vi "Get Route Distance.vi"(8 "Error In":errorcluster, 11 "ROute Index":i32) -> (0 "error out":errorcluster, 3 "Distance":dbl)   [LabVIEW 2014]
uses:
  C:/Robotic Systems/Products/AgFalcon/Software/Ground Station/Data/Mapping DLL/GMap.NET.WindowsForms.dll
  Data/Mapping DLL/GMap.NET.WindowsForms.dll
  Reference/SubVI/Main Map Control Refernce.vi
  Missions/FGVs/Current Mission Distance/Methods/Set Mission Distance.vi
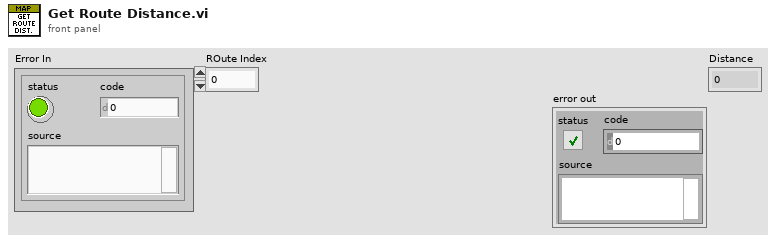
[diagram p1: front panel]
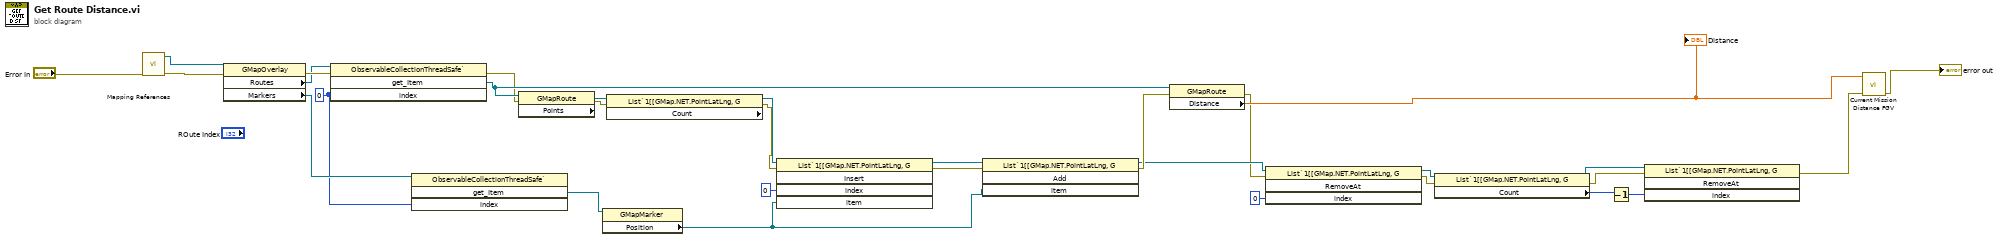
[diagram p0: block diagram]
diagram:
  w14 = 0 ("index")
  n1 = call-poly "Mapping References.vi"("Error In"="Error In") -> ("Error Out"=w30:errorcluster, "Main Map Reference"=w28:refnum<k24>)  [unwired: 9 in]
  n2 = property class="GMapOverlay"(reference=w28, error in=w30) -> (error out=w31:errorcluster, "Routes"=w29:refnum<k24>, "Markers"=w15:refnum<k24>)  [unwired: 1 out]
  n3 = invoke class="ObservableCollectionThreadSafe`" method="get_Item"(reference=w29, error in=w31, "index"=w14) -> (error out=w24:errorcluster, "get_Item"=w26:refnum<k24>)  [unwired: 1 in, 2 out]
  n4 = invoke class="ObservableCollectionThreadSafe`" method="get_Item"(reference=w15, "index"=w14) -> ("get_Item"=w13:refnum<k24>)  [unwired: 2 in, 3 out]
  n5 = property class="GMapRoute"(reference=w26, error in=w24) -> (error out=w23:errorcluster, "Points"=w25:refnum<k24>)  [unwired: 1 out]
  n6 = property class="GMapMarker"(reference=w13) -> ("Position"=w7:refnum<k24>)  [unwired: 1 in, 2 out]
  n7 = property class="List`1[[GMap.NET.PointLatLng, G" props=["Count"](reference=w25, error in=w23) -> (reference out=w20:refnum<k24>, error out=w16:errorcluster)  [unwired: 1 out]
  n8 = invoke class="List`1[[GMap.NET.PointLatLng, G" method="Insert"(reference=w20, error in=w16, "index"=0, "item"=w7) -> (reference out=w18:refnum<k24>, error out=w17:errorcluster)  [unwired: 1 in, 3 out]
  n9 = invoke class="List`1[[GMap.NET.PointLatLng, G" method="Add"(reference=w18, error in=w17, "item"=w7) -> (reference out=w11:refnum<k24>, error out=w12:errorcluster)  [unwired: 1 in, 2 out]
  n10 = property class="GMapRoute"(reference=w26, error in=w12) -> (error out=w10:errorcluster, "Distance"=w22:dbl)  [unwired: 1 out]
  "Distance" <- w22
  n11 = invoke class="List`1[[GMap.NET.PointLatLng, G" method="RemoveAt"(reference=w11, error in=w10, "index"=0) -> (reference out=w6:refnum<k24>, error out=w5:errorcluster)  [unwired: 1 in, 2 out]
  n12 = property class="List`1[[GMap.NET.PointLatLng, G"(reference=w6, error in=w5) -> (reference out=w1:refnum<k24>, error out=w2:errorcluster, "Count"=w4:i32)
  n13 = Decrement(x=w4) -> (x-1=w3:i32)
  n14 = invoke class="List`1[[GMap.NET.PointLatLng, G" method="RemoveAt"(reference=w1, error in=w2, "index"=w3) -> (error out=w9:errorcluster)  [unwired: 1 in, 3 out]
  n15 = call-poly "Current Mission Distance FGV.vi"("Error In"=w9, "Distance In (km)"=w22) -> ("Error Out"=→"error out":errorcluster)  [unwired: 9 in]
